vi "GearTipControl.vi"() -> ()   [LabVIEW 2016]
uses:
  <vilib>/Rock Robotics/WPI/Solenoid/WPI_SolenoidValue.ctl
  Robot Global Data.vi
  <vilib>/Rock Robotics/WPI/Solenoid/WPI_SolenoidSetEnum.vi
panel:
  in  "GrabCtrl":string
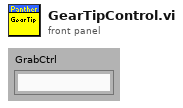
[diagram p1: front panel]
types:
  T1 = typedef "WPI_SolenoidDevRef.ctl" = cluster{"DevStatus":errorcluster, "Pneumatics Control Module":u8, "Forward Solenoid Channel":T2, "Reverse Solenoid Channel":T2}
  T2 = typedef "WPI_SolenoidChannel.ctl" = enum8{"Solenoid 0", "Solenoid 1", "Solenoid 2", "Solenoid 3", "Solenoid 4", "Solenoid 5", "Solenoid 6", "Solenoid 7", "Invalid"}
  T3 = typedef "WPI_SolenoidValue.ctl" = enum16{"Off", "On", "Forward", "Reverse"}
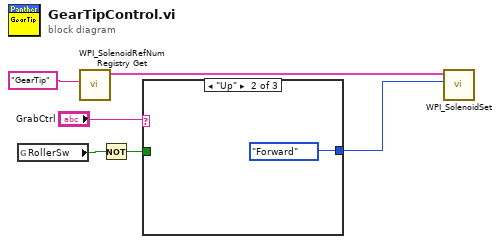
[diagram p0: block diagram]
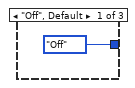
[diagram p2: hidden frame]
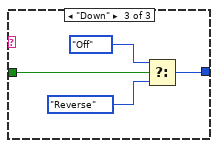
[diagram p3: hidden frame]
diagram:
  n1 = global read "Robot Global Data.vi" "RollerSw"() -> (w2:bool)
  n2 = call <vilib>:"WPI_SolenoidRefNum Registry Get.vi"("refnum name"="GearTip") -> ("SolenoidDevRef"=w4:T1)  [unwired: 1 in, 9 out]
  n3 = Not(x=w2) -> (.not. x?=w1:bool)
  n4 = case shown="\"Up\"" "GrabCtrl" {
    tunnel: [WPI_SolenoidValue."Off" ("Value") WPI_SolenoidValue."Forward" ("Value") w12] -> w6
    tunnel: w1 -> [_ _ w9]
    frame "Off", Default {
    }
    frame "Up" {
    }
    frame "Down" {
      n5 = Select(t=WPI_SolenoidValue."Off" ("Value"), s=w9, f=WPI_SolenoidValue."Reverse" ("Value")) -> (s? t:f=w12:T3)
    }
  }
  n6 = call-poly <vilib>:"WPI_SolenoidSet.vi"("Value"=w6, "SolenoidDevRef"=w4) -> ()  [unwired: 1 in, 9 out]
